vi "refs_var.vi"() -> ()   [LabVIEW 2013]
panel:
  in  "fin row ref":refnum<vi>
  in  "skip ref":refnum<vi>
  in  "stat 4 ref":refnum<vi>
  in  "stat twm ref":refnum<vi>
  in  "idn str refs":refnum<vi>[](array[refnum])
  in  "color names":string[](array[string])=["K", "W", "R", "G", "C", "O"]
  in  "colors":u32[](array[colorbox])=[0, 16448250, 16711680, 6618880, 61680, 16767232]
  in  "error ref":refnum<vi>
  in  "btn stop ref":refnum<vi>
  in  "stat 3 ref":refnum<vi>
  in  "stat 2 ref":refnum<vi>
  in  "stat 1 ref":refnum<vi>
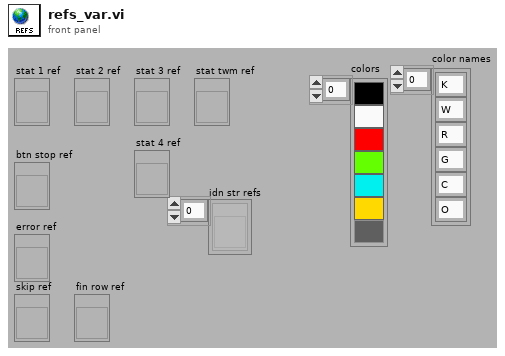
[diagram p1: front panel]
diagram:
